vi "Configure Dual Channel Phase.vi"(8 "error in (no error)":errorcluster, 9 "Phase Unwrap (T: Enable)":bool=TRUE, 10 "Analyzer (0: A0)":i32(ring) items=["A0", "A1"], 11 "VISA resource name":refnum<visa-resource-name>) -> (0 "error out":errorcluster, 3 "VISA resource name out":refnum<visa-resource-name>)   [LabVIEW 2014, in "Stanford Research SR1.lvlib"]
doc: "Configures the attributes for the Dual Channel Phase."
uses:
  Stanford Research SR1.lvlib
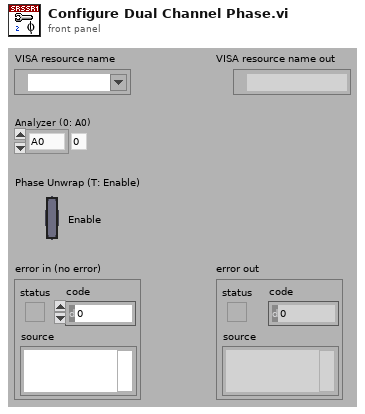
[diagram p1: front panel]
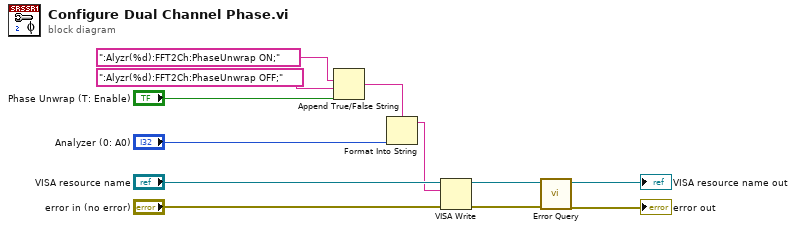
[diagram p0: block diagram]
diagram:
  n1 = Append True/False String(1:"Phase Unwrap (T: Enable)", 2:":Alyzr(%d):FFT2Ch:PhaseUnwrap OFF;", 3:":Alyzr(%d):FFT2Ch:PhaseUnwrap ON;") -> (0:w3:string)  [unwired: 1 in]
  n2 = Format Into String(format string=w3, "Analyzer (0: A0)") -> (resulting string=w1:string)  [unwired: 2 in, 1 out]
  n3 = VISA Write(VISA resource name="VISA resource name", write buffer=w1, error in (no error)="error in (no error)") -> (VISA resource name out=w7:refnum<visa-resource-name>, error out=w6:errorcluster)  [unwired: 1 out]
  n4 = call "Error Query.vi"("error in (no error)"=w6, "VISA resource name"=w7) -> ("error out"=→"error out":errorcluster, "VISA resource name out"=→"VISA resource name out":refnum<visa-resource-name>)  [unwired: 6 in, 2 out]
